vi "BMU诊断标定.vi"(5 "timeout":u32, 6 "Socket":dbl, 7 "通用配置?":bool, 8 "CAN端口":u16(ring), 9 "设备索引号":u16(ring), 10 "CAN卡类型":u32(ring)=21, 11 "从板号":u8=1) -> (3 "成功?":bool)   [LabVIEW 2013] (continued)
                      frame True {
                      }
                    }
                  }
                }
              }
            }
          }
          event "风机继电器": Value Change {
            n2723 = event-data() -> ("NewVal"=w3577:bool)  [unwired: 6 out]
            n2724 = stacked-sequence {
              tunnel: w3577 -> [_ w3590 _]
              frame #0 {
                w3581 = FALSE ("继电器超时处理")
                n2725 = local write "继电器超时处理"(w3581) -> ()
                n2726 = local write "正级继电器 6"(w3581) -> ()
                n2727 = global write "EV05全局变量1.vi" "流控帧"(FALSE ("流控帧")) -> ()
                n2728 = local write "主从选择"(enum32{"主板", "从板"}."主板" ("主从选择")) -> ()
              }
              frame #1 {
                n2729 = case shown="真" w3590 {
                  selector: w3590 -> [w3604 w3624]
                  tunnel: [w3603 w3623] -> w3589
                  tunnel: [w3592 w3612] -> w3584
                  frame True {
                    w3600 = 256.0 ("y")
                    w3592 = u32 1 ("命令序号")
                    w3603 = u8 192 ("命令")
                    n2730 = local read "动作保持时间"() -> (w3601:dbl)
                    n2731 = Quotient & Remainder(x=w3601, y=w3600) -> (x-y*floor(x/y)=w3593:dbl, floor(x/y)=w3597:dbl)
                    n2732 = Quotient & Remainder(x=w3597, y=w3600) -> (x-y*floor(x/y)=w3594:dbl, floor(x/y)=w3598:dbl)
                    n2733 = Quotient & Remainder(x=w3598, y=w3600) -> (x-y*floor(x/y)=w3595:dbl, floor(x/y)=w3599:dbl)
                    n2734 = Boolean To (0,1)(Boolean=w3604) -> (0, 1=w3602:i16)
                    n2735 = local read "设备索引号"() -> (w3609:u16)
                    n2736 = local read "CAN卡类型"() -> (w3610:u32)
                    n2737 = Quotient & Remainder(x=w3599, y=w3600) -> (x-y*floor(x/y)=w3596:dbl)  [unwired: 1 out]
                    n2738 = local read "CAN端口"() -> (w3608:u16)
                    n2739 = Build Array(i16 6 ("元素"), w3602, w3596, w3595, w3594, w3593, 0.0 ("元素")) -> (w3606:dbl[])
                    n2740 = call "多帧发送机制(EV05).vi"("can卡类型"=w3610, "设备索引号"=w3609, "CAN端口"=w3608, "命令"=w3603, "板号"=u8 0, "命令序号"=w3592, "输入数据"=w3606) -> ()  [unwired: 2 in, 11 out]
                  }
                  frame False {
                    w3620 = 256.0 ("y")
                    w3612 = u32 1 ("命令序号")
                    w3623 = u8 192 ("命令")
                    n2741 = local read "动作保持时间"() -> (w3621:dbl)
                    n2742 = Quotient & Remainder(x=w3621, y=w3620) -> (x-y*floor(x/y)=w3613:dbl, floor(x/y)=w3617:dbl)
                    n2743 = Quotient & Remainder(x=w3617, y=w3620) -> (x-y*floor(x/y)=w3614:dbl, floor(x/y)=w3618:dbl)
                    n2744 = Quotient & Remainder(x=w3618, y=w3620) -> (x-y*floor(x/y)=w3615:dbl, floor(x/y)=w3619:dbl)
                    n2745 = Boolean To (0,1)(Boolean=w3624) -> (0, 1=w3622:i16)
                    n2746 = local read "设备索引号"() -> (w3629:u16)
                    n2747 = local read "CAN卡类型"() -> (w3630:u32)
                    n2748 = Quotient & Remainder(x=w3619, y=w3620) -> (x-y*floor(x/y)=w3616:dbl)  [unwired: 1 out]
                    n2749 = local read "CAN端口"() -> (w3628:u16)
                    n2750 = Build Array(i16 6 ("元素"), w3622, w3616, w3615, w3614, w3613, 0.0 ("元素")) -> (w3626:dbl[])
                    n2751 = call "多帧发送机制(EV05).vi"("can卡类型"=w3630, "设备索引号"=w3629, "CAN端口"=w3628, "命令"=w3623, "板号"=u8 0, "命令序号"=w3612, "输入数据"=w3626) -> ()  [unwired: 2 in, 11 out]
                  }
                }
                n2752 = local write "命令序号"(w3584) -> ()
                n2753 = local write "命令"(w3589) -> ()
                n2754 = local write "清BUFF"(FALSE ("清BUFF")) -> ()
                n2755 = local write "控制1"(TRUE ("控制1")) -> ()
                n2756 = global write "EV05全局变量1.vi" "流控帧 2"(TRUE ("流控帧 2")) -> ()
                n2757 = local write "写?"(FALSE ("写?")) -> ()
                n2758 = local write "消除"(TRUE ("消除")) -> ()
              }
              frame #2 {
                n2759 = flat-sequence {
                  tunnel: [w3632] -> w3631
                  tunnel: w3631 -> [w3639]
                  frame #0 {
                    n2760 = while {
                      tunnel: [w3633] -> w3632
                      i -> [w3637]
                      stop <- w3634 stop-if-true
                      n2761 = local read "继电器超时处理"() -> (w3633:bool)
                      n2762 = Greater Or Equal?(x=w3637, y=20) -> (x >= y?=w3635:bool)
                      n2763 = Wait Until Next ms Multiple(millisecond multiple=u32 100 ("毫秒倍数")) -> ()  [unwired: 1 out]
                      n2764 = Or(x=w3633, y=w3635) -> (x .or. y?=w3634:bool)
                    }
                  }
                  frame #1 {
                    n2765 = case shown="假" w3639 {
                      frame False {
                        n2766 = local read "风机继电器"() -> (w3640:bool)
                        n2767 = Not(x=w3640) -> (.not. x?=w3641:bool)
                        n2768 = local write "风机继电器"(w3641) -> ()
                        n2769 = One Button Dialog(message="继电器处理超时" ("消息"), button name ("OK")="是" ("按钮名称（“确定”）")) -> ()  [unwired: 1 out]
                      }
                      frame True {
                      }
                    }
                  }
                }
              }
            }
          }
          event "加热继电器(从)": Value Change {
            n2770 = event-data() -> ("NewVal"=w3644:bool)  [unwired: 6 out]
            n2771 = stacked-sequence {
              tunnel: w3644 -> [_ w3658 _]
              frame #0 {
                w3648 = FALSE ("继电器超时处理")
                n2772 = local write "正级继电器 7"(w3648) -> ()
                n2773 = local write "继电器超时处理"(w3648) -> ()
                n2774 = global write "EV05全局变量1.vi" "流控帧"(FALSE ("流控帧")) -> ()
                n2775 = local write "主从选择"(enum32{"主板", "从板"}."从板" ("主从选择")) -> ()
              }
              frame #1 {
                n2776 = case shown="真" w3658 {
                  selector: w3658 -> [w3673 w3693]
                  tunnel: [w3672 w3692] -> w3657
                  tunnel: [w3671 w3691] -> w3651
                  tunnel: [w3660 w3680] -> w3652
                  frame True {
                    w3668 = 256.0 ("y")
                    w3660 = u32 1 ("命令序号")
                    w3672 = u8 192 ("命令")
                    n2777 = local read "动作保持时间"() -> (w3669:dbl)
                    n2778 = Quotient & Remainder(x=w3669, y=w3668) -> (x-y*floor(x/y)=w3661:dbl, floor(x/y)=w3665:dbl)
                    n2779 = Quotient & Remainder(x=w3665, y=w3668) -> (x-y*floor(x/y)=w3662:dbl, floor(x/y)=w3666:dbl)
                    n2780 = Quotient & Remainder(x=w3666, y=w3668) -> (x-y*floor(x/y)=w3663:dbl, floor(x/y)=w3667:dbl)
                    n2781 = Quotient & Remainder(x=w3667, y=w3668) -> (x-y*floor(x/y)=w3664:dbl)  [unwired: 1 out]
                    n2782 = Boolean To (0,1)(Boolean=w3673) -> (0, 1=w3670:i16)
                    n2783 = local read "设备索引号"() -> (w3677:u16)
                    n2784 = local read "CAN卡类型"() -> (w3678:u32)
                    n2785 = local read "从板板号"() -> (w3671:u8)
                    n2786 = local read "CAN端口"() -> (w3676:u16)
                    n2787 = Build Array(i16 7 ("元素"), w3670, w3664, w3663, w3662, w3661, 0.0 ("元素")) -> (w3675:dbl[])
                    n2788 = call "多帧发送机制(EV05).vi"("can卡类型"=w3678, "设备索引号"=w3677, "CAN端口"=w3676, "命令"=w3672, "板号"=w3671, "命令序号"=w3660, "输入数据"=w3675) -> ()  [unwired: 2 in, 11 out]
                  }
                  frame False {
                    w3688 = 256.0 ("y")
                    w3680 = u32 1 ("命令序号")
                    w3692 = u8 192 ("命令")
                    n2789 = local read "动作保持时间"() -> (w3689:dbl)
                    n2790 = Quotient & Remainder(x=w3689, y=w3688) -> (x-y*floor(x/y)=w3681:dbl, floor(x/y)=w3685:dbl)
                    n2791 = Quotient & Remainder(x=w3685, y=w3688) -> (x-y*floor(x/y)=w3682:dbl, floor(x/y)=w3686:dbl)
                    n2792 = Quotient & Remainder(x=w3686, y=w3688) -> (x-y*floor(x/y)=w3683:dbl, floor(x/y)=w3687:dbl)
                    n2793 = Quotient & Remainder(x=w3687, y=w3688) -> (x-y*floor(x/y)=w3684:dbl)  [unwired: 1 out]
                    n2794 = Boolean To (0,1)(Boolean=w3693) -> (0, 1=w3690:i16)
                    n2795 = local read "设备索引号"() -> (w3697:u16)
                    n2796 = local read "CAN卡类型"() -> (w3698:u32)
                    n2797 = local read "从板板号"() -> (w3691:u8)
                    n2798 = local read "CAN端口"() -> (w3696:u16)
                    n2799 = Build Array(i16 7 ("元素"), w3690, w3684, w3683, w3682, w3681, 0.0 ("元素")) -> (w3695:dbl[])
                    n2800 = call "多帧发送机制(EV05).vi"("can卡类型"=w3698, "设备索引号"=w3697, "CAN端口"=w3696, "命令"=w3692, "板号"=w3691, "命令序号"=w3680, "输入数据"=w3695) -> ()  [unwired: 2 in, 11 out]
                  }
                }
                n2801 = local write "从板板号"(w3651) -> ()
                n2802 = local write "命令序号"(w3652) -> ()
                n2803 = local write "命令"(w3657) -> ()
                n2804 = local write "清BUFF"(FALSE ("清BUFF")) -> ()
                n2805 = local write "写?"(FALSE ("写?")) -> ()
                n2806 = local write "控制1"(TRUE ("控制1")) -> ()
                n2807 = global write "EV05全局变量1.vi" "流控帧 2"(TRUE ("流控帧 2")) -> ()
                n2808 = local write "消除"(TRUE ("消除")) -> ()
              }
              frame #2 {
                n2809 = flat-sequence {
                  tunnel: [w3700] -> w3699
                  tunnel: w3699 -> [w3707]
                  frame #0 {
                    n2810 = while {
                      tunnel: [w3701] -> w3700
                      i -> [w3705]
                      stop <- w3702 stop-if-true
                      n2811 = local read "继电器超时处理"() -> (w3701:bool)
                      n2812 = Greater Or Equal?(x=w3705, y=20) -> (x >= y?=w3703:bool)
                      n2813 = Wait Until Next ms Multiple(millisecond multiple=u32 100 ("毫秒倍数")) -> ()  [unwired: 1 out]
                      n2814 = Or(x=w3701, y=w3703) -> (x .or. y?=w3702:bool)
                    }
                  }
                  frame #1 {
                    n2815 = case shown="假" w3707 {
                      frame False {
                        n2816 = local read "加热继电器(从)"() -> (w3709:bool)
                        n2817 = Not(x=w3709) -> (.not. x?=w3708:bool)
                        n2818 = local write "加热继电器(从)"(w3708) -> ()
                        n2819 = One Button Dialog(message="继电器处理超时" ("消息"), button name ("OK")="是" ("按钮名称（“确定”）")) -> ()  [unwired: 1 out]
                      }
                      frame True {
                      }
                    }
                  }
                }
              }
            }
          }
          event "风机继电器(从)": Value Change {
            n2820 = event-data() -> ("NewVal"=w3712:bool)  [unwired: 6 out]
            n2821 = stacked-sequence {
              tunnel: w3712 -> [_ w3726 _]
              frame #0 {
                w3716 = FALSE ("继电器超时处理")
                n2822 = local write "继电器超时处理"(w3716) -> ()
                n2823 = local write "正级继电器 8"(w3716) -> ()
                n2824 = global write "EV05全局变量1.vi" "流控帧"(FALSE ("流控帧")) -> ()
                n2825 = local write "主从选择"(enum32{"主板", "从板"}."从板" ("主从选择")) -> ()
              }
              frame #1 {
                n2826 = case shown="假" w3726 {
                  selector: w3726 -> [w3741 w3761]
                  tunnel: [w3740 w3760] -> w3725
                  tunnel: [w3739 w3759] -> w3719
                  tunnel: [w3728 w3748] -> w3720
                  frame False {
                    w3736 = 256.0 ("y")
                    w3728 = u32 1 ("命令序号")
                    w3740 = u8 192 ("命令")
                    n2827 = local read "动作保持时间"() -> (w3737:dbl)
                    n2828 = Quotient & Remainder(x=w3737, y=w3736) -> (x-y*floor(x/y)=w3729:dbl, floor(x/y)=w3733:dbl)
                    n2829 = Quotient & Remainder(x=w3733, y=w3736) -> (x-y*floor(x/y)=w3730:dbl, floor(x/y)=w3734:dbl)
                    n2830 = Quotient & Remainder(x=w3734, y=w3736) -> (x-y*floor(x/y)=w3731:dbl, floor(x/y)=w3735:dbl)
                    n2831 = Quotient & Remainder(x=w3735, y=w3736) -> (x-y*floor(x/y)=w3732:dbl)  [unwired: 1 out]
                    n2832 = local read "设备索引号"() -> (w3745:u16)
                    n2833 = local read "CAN卡类型"() -> (w3746:u32)
                    n2834 = local read "从板板号"() -> (w3739:u8)
                    n2835 = Boolean To (0,1)(Boolean=w3741) -> (0, 1=w3738:i16)
                    n2836 = local read "CAN端口"() -> (w3744:u16)
                    n2837 = Build Array(i16 8 ("元素"), w3738, w3732, w3731, w3730, w3729, 0.0 ("元素")) -> (w3743:dbl[])
                    n2838 = call "多帧发送机制(EV05).vi"("can卡类型"=w3746, "设备索引号"=w3745, "CAN端口"=w3744, "命令"=w3740, "板号"=w3739, "命令序号"=w3728, "输入数据"=w3743) -> ()  [unwired: 2 in, 11 out]
                  }
                  frame True {
                    w3756 = 256.0 ("y")
                    w3748 = u32 1 ("命令序号")
                    w3760 = u8 192 ("命令")
                    n2839 = local read "动作保持时间"() -> (w3757:dbl)
                    n2840 = Quotient & Remainder(x=w3757, y=w3756) -> (x-y*floor(x/y)=w3749:dbl, floor(x/y)=w3753:dbl)
                    n2841 = Quotient & Remainder(x=w3753, y=w3756) -> (x-y*floor(x/y)=w3750:dbl, floor(x/y)=w3754:dbl)
                    n2842 = Quotient & Remainder(x=w3754, y=w3756) -> (x-y*floor(x/y)=w3751:dbl, floor(x/y)=w3755:dbl)
                    n2843 = Quotient & Remainder(x=w3755, y=w3756) -> (x-y*floor(x/y)=w3752:dbl)  [unwired: 1 out]
                    n2844 = local read "设备索引号"() -> (w3765:u16)
                    n2845 = local read "CAN卡类型"() -> (w3766:u32)
                    n2846 = local read "从板板号"() -> (w3759:u8)
                    n2847 = Boolean To (0,1)(Boolean=w3761) -> (0, 1=w3758:i16)
                    n2848 = local read "CAN端口"() -> (w3764:u16)
                    n2849 = Build Array(i16 8 ("元素"), w3758, w3752, w3751, w3750, w3749, 0.0 ("元素")) -> (w3763:dbl[])
                    n2850 = call "多帧发送机制(EV05).vi"("can卡类型"=w3766, "设备索引号"=w3765, "CAN端口"=w3764, "命令"=w3760, "板号"=w3759, "命令序号"=w3748, "输入数据"=w3763) -> ()  [unwired: 2 in, 11 out]
                  }
                }
                n2851 = local write "从板板号"(w3719) -> ()
                n2852 = local write "清BUFF"(FALSE ("清BUFF")) -> ()
                n2853 = local write "命令序号"(w3720) -> ()
                n2854 = local write "命令"(w3725) -> ()
                n2855 = local write "控制1"(TRUE ("控制1")) -> ()
                n2856 = local write "写?"(FALSE ("写?")) -> ()
                n2857 = local write "消除"(TRUE ("消除")) -> ()
                n2858 = global write "EV05全局变量1.vi" "流控帧 2"(TRUE ("流控帧 2")) -> ()
              }
              frame #2 {
                n2859 = flat-sequence {
                  tunnel: [w3768] -> w3767
                  tunnel: w3767 -> [w3775]
                  frame #0 {
                    n2860 = while {
                      tunnel: [w3769] -> w3768
                      i -> [w3773]
                      stop <- w3770 stop-if-true
                      n2861 = local read "继电器超时处理"() -> (w3769:bool)
                      n2862 = Greater Or Equal?(x=w3773, y=20) -> (x >= y?=w3771:bool)
                      n2863 = Wait Until Next ms Multiple(millisecond multiple=u32 100 ("毫秒倍数")) -> ()  [unwired: 1 out]
                      n2864 = Or(x=w3769, y=w3771) -> (x .or. y?=w3770:bool)
                    }
                  }
                  frame #1 {
                    n2865 = case shown="假" w3775 {
                      frame False {
                        n2866 = local read "风机继电器(从)"() -> (w3777:bool)
                        n2867 = Not(x=w3777) -> (.not. x?=w3776:bool)
                        n2868 = local write "风机继电器(从)"(w3776) -> ()
                        n2869 = One Button Dialog(message="继电器处理超时" ("消息"), button name ("OK")="是" ("按钮名称（“确定”）")) -> ()  [unwired: 1 out]
                      }
                      frame True {
                      }
                    }
                  }
                }
              }
            }
          }
          event "DO1": Value Change {
            n2870 = event-data() -> ("NewVal"=w3780:bool)  [unwired: 6 out]
            n2871 = stacked-sequence {
              tunnel: w3780 -> [_ w3793 _]
              frame #0 {
                w3783 = FALSE ("清BUFF")
                n2872 = local write "继电器超时处理"(FALSE ("继电器超时处理")) -> ()
                n2873 = local write "清BUFF"(w3783) -> ()
                n2874 = local write "正级继电器 9"(w3783) -> ()
                n2875 = local write "主从选择"(enum32{"主板", "从板"}."主板" ("主从选择")) -> ()
              }
              frame #1 {
                n2876 = case shown="真" w3793 {
                  selector: w3793 -> [w3808 w3828]
                  tunnel: [w3807 w3827] -> w3792
                  tunnel: [w3795 w3815] -> w3787
                  frame False {
                    w3803 = 256.0 ("y")
                    w3795 = u32 2 ("命令序号")
                    w3807 = u8 192 ("命令")
                    n2877 = local read "动作保持时间"() -> (w3804:dbl)
                    n2878 = Quotient & Remainder(x=w3804, y=w3803) -> (x-y*floor(x/y)=w3796:dbl, floor(x/y)=w3800:dbl)
                    n2879 = Quotient & Remainder(x=w3800, y=w3803) -> (x-y*floor(x/y)=w3797:dbl, floor(x/y)=w3801:dbl)
                    n2880 = Quotient & Remainder(x=w3801, y=w3803) -> (x-y*floor(x/y)=w3798:dbl, floor(x/y)=w3802:dbl)
                    n2881 = local read "设备索引号"() -> (w3812:u16)
                    n2882 = local read "CAN卡类型"() -> (w3813:u32)
                    n2883 = local read "CAN端口"() -> (w3811:u16)
                    n2884 = Boolean To (0,1)(Boolean=w3808) -> (0, 1=w3805:i16)
                    n2885 = Quotient & Remainder(x=w3802, y=w3803) -> (x-y*floor(x/y)=w3799:dbl)  [unwired: 1 out]
                    n2886 = Build Array(i16 1 ("元素"), w3805, w3799, w3798, w3797, w3796, 0.0 ("元素")) -> (w3809:dbl[])
                    n2887 = call "多帧发送机制(EV05).vi"("can卡类型"=w3813, "设备索引号"=w3812, "CAN端口"=w3811, "命令"=w3807, "板号"=u8 0, "命令序号"=w3795, "输入数据"=w3809) -> ()  [unwired: 2 in, 11 out]
                  }
                  frame True {
                    w3823 = 256.0 ("y")
                    w3815 = u32 2 ("命令序号")
                    w3827 = u8 192 ("命令")
                    n2888 = local read "动作保持时间"() -> (w3824:dbl)
                    n2889 = Quotient & Remainder(x=w3824, y=w3823) -> (x-y*floor(x/y)=w3816:dbl, floor(x/y)=w3820:dbl)
                    n2890 = Quotient & Remainder(x=w3820, y=w3823) -> (x-y*floor(x/y)=w3817:dbl, floor(x/y)=w3821:dbl)
                    n2891 = Quotient & Remainder(x=w3821, y=w3823) -> (x-y*floor(x/y)=w3818:dbl, floor(x/y)=w3822:dbl)
                    n2892 = local read "设备索引号"() -> (w3832:u16)
                    n2893 = local read "CAN卡类型"() -> (w3833:u32)
                    n2894 = local read "CAN端口"() -> (w3831:u16)
                    n2895 = Boolean To (0,1)(Boolean=w3828) -> (0, 1=w3825:i16)
                    n2896 = Quotient & Remainder(x=w3822, y=w3823) -> (x-y*floor(x/y)=w3819:dbl)  [unwired: 1 out]
                    n2897 = Build Array(i16 1 ("元素"), w3825, w3819, w3818, w3817, w3816, 0.0 ("元素")) -> (w3829:dbl[])
                    n2898 = call "多帧发送机制(EV05).vi"("can卡类型"=w3833, "设备索引号"=w3832, "CAN端口"=w3831, "命令"=w3827, "板号"=u8 0, "命令序号"=w3815, "输入数据"=w3829) -> ()  [unwired: 2 in, 11 out]
                  }
                }
                n2899 = local write "命令序号"(w3787) -> ()
                n2900 = local write "命令"(w3792) -> ()
                n2901 = local write "控制1"(TRUE ("控制1")) -> ()
                n2902 = local write "写?"(FALSE ("写?")) -> ()
                n2903 = local write "消除"(TRUE ("消除")) -> ()
                n2904 = global write "EV05全局变量1.vi" "流控帧 2"(TRUE ("流控帧 2")) -> ()
                n2905 = global write "EV05全局变量1.vi" "流控帧"(FALSE ("流控帧")) -> ()
              }
              frame #2 {
                n2906 = flat-sequence {
                  tunnel: [w3835] -> w3834
                  tunnel: w3834 -> [w3842]
                  frame #0 {
                    n2907 = while {
                      tunnel: [w3836] -> w3835
                      i -> [w3840]
                      stop <- w3837 stop-if-true
                      n2908 = local read "继电器超时处理"() -> (w3836:bool)
                      n2909 = Greater Or Equal?(x=w3840, y=20) -> (x >= y?=w3838:bool)
                      n2910 = Wait Until Next ms Multiple(millisecond multiple=u32 100 ("毫秒倍数")) -> ()  [unwired: 1 out]
                      n2911 = Or(x=w3836, y=w3838) -> (x .or. y?=w3837:bool)
                    }
                  }
                  frame #1 {
                    n2912 = case shown="假" w3842 {
                      frame False {
                        n2913 = local read "DO1"() -> (w3844:bool)
                        n2914 = Not(x=w3844) -> (.not. x?=w3843:bool)
                        n2915 = local write "DO1"(w3843) -> ()
                        n2916 = One Button Dialog(message="DO控制处理超时" ("消息"), button name ("OK")="是" ("按钮名称（“确定”）")) -> ()  [unwired: 1 out]
                      }
                      frame True {
                      }
                    }
                  }
                }
              }
            }
          }
          event "DO2": Value Change {
            n2917 = event-data() -> ("NewVal"=w3847:bool)  [unwired: 6 out]
            n2918 = stacked-sequence {
              tunnel: w3847 -> [_ w3860 _]
              frame #0 {
                w3850 = FALSE ("清BUFF")
                n2919 = local write "继电器超时处理"(FALSE ("继电器超时处理")) -> ()
                n2920 = local write "主从选择"(enum32{"主板", "从板"}."主板" ("主从选择")) -> ()
                n2921 = local write "清BUFF"(w3850) -> ()
                n2922 = local write "正级继电器 10"(w3850) -> ()
              }
              frame #1 {
                n2923 = case shown="真" w3860 {
                  selector: w3860 -> [w3875 w3895]
                  tunnel: [w3874 w3894] -> w3859
                  tunnel: [w3862 w3882] -> w3854
                  frame False {
                    w3870 = 256.0 ("y")
                    w3862 = u32 2 ("命令序号")
                    w3874 = u8 192 ("命令")
                    n2924 = local read "动作保持时间"() -> (w3871:dbl)
                    n2925 = Quotient & Remainder(x=w3871, y=w3870) -> (x-y*floor(x/y)=w3863:dbl, floor(x/y)=w3867:dbl)
                    n2926 = Quotient & Remainder(x=w3867, y=w3870) -> (x-y*floor(x/y)=w3864:dbl, floor(x/y)=w3868:dbl)
                    n2927 = Quotient & Remainder(x=w3868, y=w3870) -> (x-y*floor(x/y)=w3865:dbl, floor(x/y)=w3869:dbl)
                    n2928 = local read "设备索引号"() -> (w3879:u16)
                    n2929 = local read "CAN卡类型"() -> (w3880:u32)
                    n2930 = local read "CAN端口"() -> (w3878:u16)
                    n2931 = Boolean To (0,1)(Boolean=w3875) -> (0, 1=w3872:i16)
                    n2932 = Quotient & Remainder(x=w3869, y=w3870) -> (x-y*floor(x/y)=w3866:dbl)  [unwired: 1 out]
                    n2933 = Build Array(i16 2 ("元素"), w3872, w3866, w3865, w3864, w3863, 0.0 ("元素")) -> (w3876:dbl[])
                    n2934 = call "多帧发送机制(EV05).vi"("can卡类型"=w3880, "设备索引号"=w3879, "CAN端口"=w3878, "命令"=w3874, "板号"=u8 0, "命令序号"=w3862, "输入数据"=w3876) -> ()  [unwired: 2 in, 11 out]
                  }
                  frame True {
                    w3890 = 256.0 ("y")
                    w3882 = u32 2 ("命令序号")
                    w3894 = u8 192 ("命令")
                    n2935 = local read "动作保持时间"() -> (w3891:dbl)
                    n2936 = Quotient & Remainder(x=w3891, y=w3890) -> (x-y*floor(x/y)=w3883:dbl, floor(x/y)=w3887:dbl)
                    n2937 = Quotient & Remainder(x=w3887, y=w3890) -> (x-y*floor(x/y)=w3884:dbl, floor(x/y)=w3888:dbl)
                    n2938 = Quotient & Remainder(x=w3888, y=w3890) -> (x-y*floor(x/y)=w3885:dbl, floor(x/y)=w3889:dbl)
                    n2939 = local read "设备索引号"() -> (w3899:u16)
                    n2940 = local read "CAN卡类型"() -> (w3900:u32)
                    n2941 = local read "CAN端口"() -> (w3898:u16)
                    n2942 = Boolean To (0,1)(Boolean=w3895) -> (0, 1=w3892:i16)
                    n2943 = Quotient & Remainder(x=w3889, y=w3890) -> (x-y*floor(x/y)=w3886:dbl)  [unwired: 1 out]
                    n2944 = Build Array(i16 2 ("元素"), w3892, w3886, w3885, w3884, w3883, 0.0 ("元素")) -> (w3896:dbl[])
                    n2945 = call "多帧发送机制(EV05).vi"("can卡类型"=w3900, "设备索引号"=w3899, "CAN端口"=w3898, "命令"=w3894, "板号"=u8 0, "命令序号"=w3882, "输入数据"=w3896) -> ()  [unwired: 2 in, 11 out]
                  }
                }
                n2946 = local write "命令序号"(w3854) -> ()
                n2947 = local write "命令"(w3859) -> ()
                n2948 = local write "控制1"(TRUE ("控制1")) -> ()
                n2949 = local write "写?"(FALSE ("写?")) -> ()
                n2950 = local write "消除"(TRUE ("消除")) -> ()
                n2951 = global write "EV05全局变量1.vi" "流控帧 2"(TRUE ("流控帧 2")) -> ()
                n2952 = global write "EV05全局变量1.vi" "流控帧"(FALSE ("流控帧")) -> ()
              }
              frame #2 {
                n2953 = flat-sequence {
                  tunnel: [w3902] -> w3901
                  tunnel: w3901 -> [w3909]
                  frame #0 {
                    n2954 = while {
                      tunnel: [w3903] -> w3902
                      i -> [w3907]
                      stop <- w3904 stop-if-true
                      n2955 = local read "继电器超时处理"() -> (w3903:bool)
                      n2956 = Greater Or Equal?(x=w3907, y=20) -> (x >= y?=w3905:bool)
                      n2957 = Wait Until Next ms Multiple(millisecond multiple=u32 100 ("毫秒倍数")) -> ()  [unwired: 1 out]
                      n2958 = Or(x=w3903, y=w3905) -> (x .or. y?=w3904:bool)
                    }
                  }
                  frame #1 {
                    n2959 = case shown="假" w3909 {
                      frame False {
                        n2960 = local read "DO2"() -> (w3911:bool)
                        n2961 = Not(x=w3911) -> (.not. x?=w3910:bool)
                        n2962 = local write "DO2"(w3910) -> ()
                        n2963 = One Button Dialog(message="DO控制处理超时" ("消息"), button name ("OK")="是" ("按钮名称（“确定”）")) -> ()  [unwired: 1 out]
                      }
                      frame True {
                      }
                    }
                  }
                }
              }
            }
          }
          event "DO1 2": Value Change {
            n2964 = event-data() -> ("NewVal"=w3914:bool)  [unwired: 6 out]
            n2965 = stacked-sequence {
              tunnel: w3914 -> [_ w3928 _]
              frame #0 {
                w3917 = FALSE ("继电器超时处理")
                n2966 = local write "继电器超时处理"(w3917) -> ()
                n2967 = local write "正级继电器 11"(w3917) -> ()
                n2968 = local write "主从选择"(enum32{"主板", "从板"}."从板" ("主从选择")) -> ()
              }
              frame #1 {
                n2969 = case shown="假" w3928 {
                  selector: w3928 -> [w3943 w3963]
                  tunnel: [w3942 w3962] -> w3927
                  tunnel: [w3941 w3961] -> w3921
                  tunnel: [w3930 w3950] -> w3922
                  frame True {
                    w3938 = 256.0 ("y")
                    w3930 = u32 2 ("命令序号")
                    w3942 = u8 192 ("命令")
                    n2970 = local read "动作保持时间"() -> (w3939:dbl)
                    n2971 = Quotient & Remainder(x=w3939, y=w3938) -> (x-y*floor(x/y)=w3931:dbl, floor(x/y)=w3935:dbl)
                    n2972 = Quotient & Remainder(x=w3935, y=w3938) -> (x-y*floor(x/y)=w3932:dbl, floor(x/y)=w3936:dbl)
                    n2973 = Quotient & Remainder(x=w3936, y=w3938) -> (x-y*floor(x/y)=w3933:dbl, floor(x/y)=w3937:dbl)
                    n2974 = Quotient & Remainder(x=w3937, y=w3938) -> (x-y*floor(x/y)=w3934:dbl)  [unwired: 1 out]
                    n2975 = Boolean To (0,1)(Boolean=w3943) -> (0, 1=w3940:i16)
                    n2976 = local read "设备索引号"() -> (w3947:u16)
                    n2977 = local read "CAN卡类型"() -> (w3948:u32)
                    n2978 = local read "从板板号"() -> (w3941:u8)
                    n2979 = local read "CAN端口"() -> (w3946:u16)
                    n2980 = Build Array(i16 3 ("元素"), w3940, w3934, w3933, w3932, w3931, 0.0 ("元素")) -> (w3945:dbl[])
                    n2981 = call "多帧发送机制(EV05).vi"("can卡类型"=w3948, "设备索引号"=w3947, "CAN端口"=w3946, "命令"=w3942, "板号"=w3941, "命令序号"=w3930, "输入数据"=w3945) -> ()  [unwired: 2 in, 11 out]
                  }
                  frame False {
                    w3958 = 256.0 ("y")
                    w3950 = u32 2 ("命令序号")
                    w3962 = u8 192 ("命令")
                    n2982 = local read "动作保持时间"() -> (w3959:dbl)
                    n2983 = Quotient & Remainder(x=w3959, y=w3958) -> (x-y*floor(x/y)=w3951:dbl, floor(x/y)=w3955:dbl)
                    n2984 = Quotient & Remainder(x=w3955, y=w3958) -> (x-y*floor(x/y)=w3952:dbl, floor(x/y)=w3956:dbl)
                    n2985 = Quotient & Remainder(x=w3956, y=w3958) -> (x-y*floor(x/y)=w3953:dbl, floor(x/y)=w3957:dbl)
                    n2986 = Quotient & Remainder(x=w3957, y=w3958) -> (x-y*floor(x/y)=w3954:dbl)  [unwired: 1 out]
                    n2987 = Boolean To (0,1)(Boolean=w3963) -> (0, 1=w3960:i16)
                    n2988 = local read "设备索引号"() -> (w3967:u16)
                    n2989 = local read "CAN卡类型"() -> (w3968:u32)
                    n2990 = local read "从板板号"() -> (w3961:u8)
                    n2991 = local read "CAN端口"() -> (w3966:u16)
                    n2992 = Build Array(i16 1 ("元素"), w3960, w3954, w3953, w3952, w3951, 0.0 ("元素")) -> (w3965:dbl[])
                    n2993 = call "多帧发送机制(EV05).vi"("can卡类型"=w3968, "设备索引号"=w3967, "CAN端口"=w3966, "命令"=w3962, "板号"=w3961, "命令序号"=w3950, "输入数据"=w3965) -> ()  [unwired: 2 in, 11 out]
                  }
                }
                n2994 = local write "从板板号"(w3921) -> ()
                n2995 = local write "命令序号"(w3922) -> ()
                n2996 = local write "命令"(w3927) -> ()
                n2997 = local write "清BUFF"(FALSE ("清BUFF")) -> ()
                n2998 = local write "写?"(FALSE ("写?")) -> ()
                n2999 = local write "控制1"(TRUE ("控制1")) -> ()
                n3000 = global write "EV05全局变量1.vi" "流控帧"(FALSE ("流控帧")) -> ()
                n3001 = global write "EV05全局变量1.vi" "流控帧 2"(TRUE ("流控帧 2")) -> ()
                n3002 = local write "消除"(TRUE ("消除")) -> ()
              }
              frame #2 {
                n3003 = flat-sequence {
                  tunnel: [w3970] -> w3969
                  tunnel: w3969 -> [w3977]
                  frame #0 {
                    n3004 = while {
                      tunnel: [w3971] -> w3970
                      i -> [w3975]
                      stop <- w3972 stop-if-true
                      n3005 = local read "继电器超时处理"() -> (w3971:bool)
                      n3006 = Greater Or Equal?(x=w3975, y=20) -> (x >= y?=w3973:bool)
                      n3007 = Wait Until Next ms Multiple(millisecond multiple=u32 100 ("毫秒倍数")) -> ()  [unwired: 1 out]
                      n3008 = Or(x=w3971, y=w3973) -> (x .or. y?=w3972:bool)
                    }
                  }
                  frame #1 {
                    n3009 = case shown="假" w3977 {
                      frame False {
                        n3010 = local read "DO1 2"() -> (w3979:bool)
                        n3011 = Not(x=w3979) -> (.not. x?=w3978:bool)
                        n3012 = local write "DO1 2"(w3978) -> ()
                        n3013 = One Button Dialog(message="DO控制处理超时" ("消息"), button name ("OK")="是" ("按钮名称（“确定”）")) -> ()  [unwired: 1 out]
                      }
                      frame True {
                      }
                    }
                  }
                }
              }
            }
          }
          event "读取转换为写入": Value Change {
            n3014 = event-data() -> ("NewVal"=w3982:bool)  [unwired: 6 out]
            n3015 = case shown="真" w3982 {
              tunnel: w3986 -> [w3988 w3993]
              tunnel: [w3988 w3992] -> w3985
              tunnel: w3984 -> [w3987 w3991]
              tunnel: [w3987 w3990] -> w3983
              frame False {
              }
              frame True {
                n3016 = Enqueue Element(queue=w3993, element="读取转换为写入", error in (no error)=w3991) -> (queue out=w3992:refnum<queue>, error out=w3990:errorcluster)  [unwired: 2 out]
              }
            }
          }
          event "读取故障详细状态": Value Change {
            n3017 = event-data() -> ("NewVal"=w3998:bool)  [unwired: 5 out]
            n3018 = case shown="真" w3998 {
              tunnel: w3997 -> [w4000 w4013]
              tunnel: w3996 -> [w3999 w4012]
              tunnel: [w4000 w4011] -> w3995
              tunnel: [w3999 w4010] -> w3994
              frame False {
              }
              frame True {
                n3019 = disable-structure shown="启用" {
                  disable-tunnel: [w4022 TRUE ("发送成功")] -> w4009
                  frame Disabled {
                    n3020 = local read "主从选择"() -> (w4014:enum32{"主板", "从板"})
                    n3021 = case shown="\"主板\", 默认" w4014 {
                      tunnel: [0.0 ("FUNC") w4024] -> w4019
                      frame "主板", Default {
                      }
                      frame "从板" {
                        n3022 = local read "从板号"() -> (w4024:u8)
                      }
                    }
                    n3023 = local read "设备索引号"() -> (w4016:u16)
                    n3024 = local read "CAN卡类型"() -> (w4017:u32)
                    n3025 = local read "CAN端口"() -> (w4015:u16)
                    n3026 = call "标定授权发送.vi"("CAN卡类型"=w4017, "解锁类型"=enum16{"读取", "写", "下载"}."写", "设备索引号"=w4016, "CAN端口"=w4015, "是否连接"=TRUE, "板选择"=0, "FUNC"=w4019) -> ("发送成功"=w4022:bool)  [unwired: 8 out]
                  }
                  frame Enabled {
                  }
                }
                n3027 = case shown="真" w4009 {
                  tunnel: w4013 -> [w4027 w4032]
                  tunnel: w4012 -> [w4026 w4031]
                  tunnel: [w4027 w4029] -> w4011
                  tunnel: [w4026 w4028] -> w4010
                  frame False {
                  }
                  frame True {
                    n3028 = Enqueue Element(queue=w4032, element="读取故障状态" ("元素"), error in (no error)=w4031) -> (queue out=w4029:refnum<queue>, error out=w4028:errorcluster)  [unwired: 2 out]
                  }
                }
                n3029 = local write "电池故障"(string[][] []) -> ()
                n3030 = global write "EV05全局变量1.vi" "流控帧 2"(TRUE ("流控帧")) -> ()
                n3031 = local write "写?"(FALSE ("写?")) -> ()
                n3032 = local write "控制1"(TRUE ("控制1")) -> ()
                n3033 = local write "消除"(TRUE ("消除")) -> ()
                n3034 = local write "清BUFF"(FALSE ("清BUFF")) -> ()
                n3035 = global write "EV05全局变量1.vi" "流控帧"(FALSE ("流控帧")) -> ()
                n3036 = call <vilib>:"Set Busy.vi"("disable click? (T)"=FALSE) -> ()  [unwired: 3 in, 8 out]
              }
            }
          }
          event "项目软本读取": Value Change {
            n3037 = event-data() -> ("NewVal"=w4037:bool)  [unwired: 5 out]
            n3038 = case shown="真" w4037 {
              tunnel: w4036 -> [w4039 w4046]
              tunnel: w4035 -> [w4038 w4045]
              tunnel: [w4039 w4044] -> w4034
              tunnel: [w4038 w4043] -> w4033
              frame False {
              }
              frame True {
                n3039 = global read "EV05全局变量1.vi" "授权功能"() -> (w4041:bool)
                n3040 = case shown="假" w4041 {
                  tunnel: [TRUE ("发送成功") w4065] -> w4042
                  frame False {
                  }
                  frame True {
                    n3041 = local read "设备索引号"() -> (w4060:u16)
                    n3042 = local read "CAN卡类型"() -> (w4061:u32)
                    n3043 = local read "CAN端口"() -> (w4059:u16)
                    n3044 = call "标定授权发送.vi"("CAN卡类型"=w4061, "解锁类型"=enum16{"读取", "写", "下载"}."读取", "设备索引号"=w4060, "CAN端口"=w4059, "是否连接"=TRUE, "板选择"=0, "FUNC"=u32 0) -> ("发送成功"=w4065:bool)  [unwired: 8 out]
                  }
                }
                n3045 = stacked-sequence {
                  tunnel: [w4049] -> w4040
                  frame #0 {
                    w4049 = FALSE ("disable click? (T)")
                    w4052 = FALSE ("写?")
                    n3046 = local write "写?"(w4052) -> ()
                    n3047 = global write "EV05全局变量1.vi" "写入超时"(w4052) -> ()
                    n3048 = local write "项目软件版本号"(" " ("项目软件版本号")) -> ()
                    n3049 = global write "EV05全局变量1.vi" "流控帧"(FALSE ("流控帧")) -> ()
                    n3050 = local write "主从选择"(enum32{"主板", "从板"}."主板" ("主从选择")) -> ()
                    n3051 = call <vilib>:"Set Busy.vi"("disable click? (T)"=w4049) -> ()  [unwired: 3 in, 8 out]
                    n3052 = local write "清BUFF"(FALSE ("清BUFF")) -> ()
                    n3053 = property on="保存版本信息" class="Bool (严格)"("Visible"=TRUE ("可见")) -> ()  [unwired: 2 in, 2 out]
                    n3054 = global write "EV05全局变量1.vi" "流控帧 2"(TRUE ("流控帧 2")) -> ()
                    n3055 = local write "控制1"(TRUE ("控制1")) -> ()
                    n3056 = local write "消除"(TRUE ("消除")) -> ()
                  }
                }
                n3057 = case shown="真" w4042 {
                  tunnel: w4046 -> [w4067 w4072]
                  tunnel: w4045 -> [w4066 w4071]
                  tunnel: [w4067 w4069] -> w4044
                  tunnel: [w4066 w4068] -> w4043
                  tunnel: w4040 -> [_ _]
                  frame False {
                  }
                  frame True {
                    n3058 = Enqueue Element(queue=w4072, element="项目软件版本读取" ("元素"), error in (no error)=w4071) -> (queue out=w4069:refnum<queue>, error out=w4068:errorcluster)  [unwired: 2 out]
                  }
                }
              }
            }
          }
          event "读硬件版本号": Value Change {
            n3059 = event-data() -> ("NewVal"=w4077:bool)  [unwired: 5 out]
            n3060 = case shown="真" w4077 {
              tunnel: w4076 -> [w4079 w4086]
              tunnel: w4075 -> [w4078 w4085]
              tunnel: [w4079 w4084] -> w4074
              tunnel: [w4078 w4083] -> w4073
              frame False {
              }
              frame True {
                n3061 = global read "EV05全局变量1.vi" "授权功能"() -> (w4081:bool)
                n3062 = case shown="假" w4081 {
                  tunnel: [TRUE ("发送成功") w4105] -> w4082
                  frame False {
                  }
                  frame True {
                    n3063 = local read "设备索引号"() -> (w4100:u16)
                    n3064 = local read "CAN卡类型"() -> (w4101:u32)
                    n3065 = local read "CAN端口"() -> (w4099:u16)
                    n3066 = call "标定授权发送.vi"("CAN卡类型"=w4101, "解锁类型"=enum16{"读取", "写", "下载"}."读取", "设备索引号"=w4100, "CAN端口"=w4099, "是否连接"=TRUE, "板选择"=0, "FUNC"=u32 0) -> ("发送成功"=w4105:bool)  [unwired: 8 out]
                  }
                }
                n3067 = stacked-sequence {
                  tunnel: [w4089] -> w4080
                  frame #0 {
                    w4089 = TRUE ("控制1")
                    w4093 = FALSE ("写?")
                    n3068 = local write "写?"(w4093) -> ()
                    n3069 = global write "EV05全局变量1.vi" "写入超时"(w4093) -> ()
                    n3070 = call <vilib>:"Set Busy.vi"("disable click? (T)"=FALSE) -> ()  [unwired: 3 in, 8 out]
                    n3071 = local write "硬件版本号"("" ("硬件版本号")) -> ()
                    n3072 = property on="保存版本信息" class="Bool (严格)"("Visible"=TRUE ("可见")) -> ()  [unwired: 2 in, 2 out]
                    n3073 = local write "主从选择"(enum32{"主板", "从板"}."主板" ("主从选择")) -> ()
                    n3074 = local write "控制1"(w4089) -> ()
                    n3075 = local write "清BUFF"(FALSE ("清BUFF")) -> ()
                    n3076 = global write "EV05全局变量1.vi" "流控帧 2"(TRUE ("流控帧 2")) -> ()
                    n3077 = local write "消除"(TRUE ("消除")) -> ()
                    n3078 = global write "EV05全局变量1.vi" "流控帧"(FALSE ("流控帧")) -> ()
                  }
                }
                n3079 = case shown="真" w4082 {
                  tunnel: w4086 -> [w4107 w4112]
                  tunnel: w4085 -> [w4106 w4111]
                  tunnel: [w4107 w4109] -> w4084
                  tunnel: [w4106 w4108] -> w4083
                  tunnel: w4080 -> [_ _]
                  frame False {
                  }
                  frame True {
                    n3080 = Enqueue Element(queue=w4112, element="硬件版本读取" ("元素"), error in (no error)=w4111) -> (queue out=w4109:refnum<queue>, error out=w4108:errorcluster)  [unwired: 2 out]
                  }
                }
              }
            }
          }
          event "平台软件版本读取": Value Change {
            n3081 = event-data() -> ("NewVal"=w4117:bool)  [unwired: 5 out]
            n3082 = case shown="真" w4117 {
              tunnel: w4116 -> [w4119 w4126]
              tunnel: w4115 -> [w4118 w4125]
              tunnel: [w4119 w4124] -> w4114
              tunnel: [w4118 w4123] -> w4113
              frame False {
              }
              frame True {
                n3083 = global read "EV05全局变量1.vi" "授权功能"() -> (w4121:bool)
                n3084 = case shown="假" w4121 {
                  tunnel: [TRUE ("发送成功") w4145] -> w4122
                  frame False {
                  }
                  frame True {
                    n3085 = local read "设备索引号"() -> (w4140:u16)
                    n3086 = local read "CAN卡类型"() -> (w4141:u32)
                    n3087 = local read "CAN端口"() -> (w4139:u16)
                    n3088 = call "标定授权发送.vi"("CAN卡类型"=w4141, "解锁类型"=enum16{"读取", "写", "下载"}."读取", "设备索引号"=w4140, "CAN端口"=w4139, "是否连接"=TRUE, "板选择"=0, "FUNC"=u32 0) -> ("发送成功"=w4145:bool)  [unwired: 8 out]
                  }
                }
                n3089 = stacked-sequence {
                  tunnel: [w4129] -> w4120
                  frame #0 {
                    w4129 = TRUE ("控制1")
                    w4133 = FALSE ("写?")
                    n3090 = call <vilib>:"Set Busy.vi"("disable click? (T)"=FALSE) -> ()  [unwired: 3 in, 8 out]
                    n3091 = local write "写?"(w4133) -> ()
                    n3092 = global write "EV05全局变量1.vi" "写入超时"(w4133) -> ()
                    n3093 = local write "平台软件版本号"(" " ("平台软件版本号")) -> ()
                    n3094 = local write "控制1"(w4129) -> ()
                    n3095 = local write "消除"(TRUE ("消除")) -> ()
                    n3096 = property on="保存版本信息" class="Bool (严格)"("Visible"=TRUE ("可见")) -> ()  [unwired: 2 in, 2 out]
                    n3097 = global write "EV05全局变量1.vi" "流控帧 2"(TRUE ("流控帧 2")) -> ()
                    n3098 = local write "主从选择"(enum32{"主板", "从板"}."主板" ("主从选择")) -> ()
                    n3099 = local write "清BUFF"(FALSE ("清BUFF")) -> ()
                    n3100 = global write "EV05全局变量1.vi" "流控帧"(FALSE ("流控帧")) -> ()
                  }
                }
                n3101 = case shown="真" w4122 {
                  tunnel: w4126 -> [w4147 w4152]
                  tunnel: w4125 -> [w4146 w4151]
                  tunnel: [w4147 w4149] -> w4124
                  tunnel: [w4146 w4148] -> w4123
                  tunnel: w4120 -> [_ _]
                  frame False {
                  }
                  frame True {
                    n3102 = Enqueue Element(queue=w4152, element="平台软件版本读取" ("元素"), error in (no error)=w4151) -> (queue out=w4149:refnum<queue>, error out=w4148:errorcluster)  [unwired: 2 out]
                  }
                }
              }
            }
          }
          event "模块版本读取": Value Change {
            n3103 = event-data() -> ("NewVal"=w4157:bool)  [unwired: 5 out]
            n3104 = case shown="真" w4157 {
              tunnel: w4156 -> [w4159 w4166]
              tunnel: w4155 -> [w4158 w4165]
              tunnel: [w4159 w4164] -> w4154
              tunnel: [w4158 w4163] -> w4153
              frame False {
              }
              frame True {
                n3105 = global read "EV05全局变量1.vi" "授权功能"() -> (w4161:bool)
                n3106 = case shown="假" w4161 {
                  tunnel: [TRUE ("发送成功") w4184] -> w4162
                  frame False {
                  }
                  frame True {
                    n3107 = local read "设备索引号"() -> (w4179:u16)
                    n3108 = local read "CAN卡类型"() -> (w4180:u32)
                    n3109 = local read "CAN端口"() -> (w4178:u16)
                    n3110 = call "标定授权发送.vi"("CAN卡类型"=w4180, "解锁类型"=enum16{"读取", "写", "下载"}."读取", "设备索引号"=w4179, "CAN端口"=w4178, "是否连接"=TRUE, "板选择"=0, "FUNC"=u32 0) -> ("发送成功"=w4184:bool)  [unwired: 8 out]
                  }
                }
                n3111 = stacked-sequence {
                  tunnel: [w4169] -> w4160
                  frame #0 {
                    w4169 = TRUE ("控制1")
                    w4172 = FALSE ("写?")
                    n3112 = call <vilib>:"Set Busy.vi"("disable click? (T)"=FALSE) -> ()  [unwired: 3 in, 8 out]
                    n3113 = local write "写?"(w4172) -> ()
                    n3114 = global write "EV05全局变量1.vi" "写入超时"(w4172) -> ()
                    n3115 = local write "主从选择"(enum32{"主板", "从板"}."主板" ("主从选择")) -> ()
                    n3116 = local write "清BUFF"(FALSE ("清BUFF")) -> ()
                    n3117 = property on="保存版本信息" class="Bool (严格)"("Visible"=TRUE ("可见")) -> ()  [unwired: 2 in, 2 out]
                    n3118 = global write "EV05全局变量1.vi" "流控帧 2"(TRUE ("流控帧 2")) -> ()
                    n3119 = local write "控制1"(w4169) -> ()
                    n3120 = local write "消除"(TRUE ("消除")) -> ()
                    n3121 = global write "EV05全局变量1.vi" "流控帧"(FALSE ("流控帧")) -> ()
                  }
                }
                n3122 = case shown="真" w4162 {
                  tunnel: w4166 -> [w4186 w4191]
                  tunnel: w4165 -> [w4185 w4190]
                  tunnel: [w4186 w4188] -> w4164
                  tunnel: [w4185 w4187] -> w4163
                  tunnel: w4160 -> [_ _]
                  frame False {
                  }
                  frame True {
                    n3123 = Enqueue Element(queue=w4191, element="模块软件版本读取" ("元素"), error in (no error)=w4190) -> (queue out=w4188:refnum<queue>, error out=w4187:errorcluster)  [unwired: 2 out]
                  }
                }
              }
            }
          }
          event "保存版本信息": Value Change {
            n3124 = event-data() -> ("NewVal"=w4192:bool)  [unwired: 6 out]
            n3125 = case shown="真" w4192 {
              frame False {
              }
              frame True {
                n3126 = stacked-sequence {
                  seq-local: [w4196 _] -> [_ w4198]
                  seq-local: [w4195 _] -> [_ w4197]
                  frame #0 {
                    n3127 = call "请输入从板个数"() -> ("从板个数"=w4196:dbl, "确定"=w4195:bool)  [unwired: 17 in, 1 out]
                  }
                  frame #1 {
                    n3128 = case shown="真" w4197 {
                      tunnel: w4198 -> [_ w4201]
                      frame False {
                      }
                      frame True {
                        n3129 = call <vilib>:"Application Directory.vi"() -> ("Application Directory"=w4213:path)
                        n3130 = Build Path(base path=w4213, name or relative path="SaveData" ("名称或相对路径")) -> (appended path=w4211:path)
                        n3131 = local read "模块版本名称"() -> (w4206:string[][])
                        n3132 = local read "项目软件版本"() -> (w4203:string[])
                        n3133 = local read "模块版本值"() -> (w4205:string[][])
                        n3134 = local read "平台软件版本"() -> (w4202:string[])
                        n3135 = local read "模块个数"() -> (w4199:u8[])
                        n3136 = local read "硬件版本"() -> (w4204:string[])
                        n3137 = call "文件对话框3"("start path"=w4211, "prompt"="选择要保存数据的位置", "default name"="BMS版本信息.txt") -> ("selected path"=w4207:path, "cancelled"=w4208:bool)  [unwired: 9 in, 2 out]
                        n3138 = Increment(x=w4201) -> (x+1=w4200:dbl)
                        n3139 = for {
                          N: w4200 -> [_]
                          tunnel: w4208 -> [w4229]
                          tunnel: w4207 -> [w4228]
                          tunnel: w4206 -> [w4218] mode=indexing
                          tunnel: w4205 -> [w4216] mode=indexing
                          tunnel: w4204 -> [w4223] mode=indexing
                          tunnel: w4203 -> [w4222] mode=indexing
                          tunnel: w4202 -> [w4221] mode=indexing
                          tunnel: w4199 -> [w4214] mode=indexing
                          i -> [w4220]
                          w4226 = ""
                          w4233 = 0 ("索引")
                          n3140 = case shown="0, 默认" w4220 {
                            selector: w4220 -> [_ w4247]
                            tunnel: ["主板版本信息" w4248] -> w4238
                            tunnel: [FALSE TRUE] -> w4224
                            frame 0, Default {
                            }
                            frame 1.. {
                              n3141 = Number To Decimal String(number=w4247) -> (decimal integer string=w4246:string)  [unwired: 1 in]
                              n3142 = Concatenate Strings("从板", w4246, "版本信息") -> (w4248:string)
                            }
                          }
                          n3143 = Increment(x=w4214) -> (x+1=w4215:u8)
                          n3144 = Array Subset(array=w4218, length=w4215) -> (w4219:string[])  [unwired: 1 in]
                          n3145 = Array Subset(array=w4216, length=w4215) -> (w4217:string[])  [unwired: 1 in]
                          n3146 = Build Array(w4226, w4221, w4222, w4223, w4226) -> (w4232:string[])
                          n3147 = Build Array(w4238, "平台软件版本号", "项目软件版本号", "硬件版本号", "模块版本号") -> (w4234:string[])
                          n3148 = Insert Into Array(array=w4219, index=w4233, new element=w4234) -> (w4231:string[])
                          n3149 = Insert Into Array(array=w4217, index=w4233, new element=w4232) -> (w4230:string[])
                          n3150 = Build Array(w4231, w4230) -> (w4227:string[][])
                          n3151 = case shown="假" w4229 {
                            tunnel: w4228 -> [w4242 _]
                            tunnel: w4227 -> [w4241 _]
                            tunnel: w4224 -> [w4239 _]
                            frame False {
                              n3152 = call-poly <vilib>:"Write To Spreadsheet File.vi"("transpose? (no:F)"=TRUE, "append to file? (new file:F)"=w4239, "2D data"=w4241, "file path (dialog if empty)"=w4242) -> ()  [unwired: 4 in, 1 out]
                            }
                            frame True {
                            }
                          }
                        }
                      }
                    }
                  }
                }
              }
            }
          }
          event "单个写入": Value Change {
            n3153 = event-data() -> ("NewVal"=w4255:bool)  [unwired: 5 out]
            n3154 = case shown="真" w4255 {
              tunnel: w4254 -> [w4257 w4264]
              tunnel: w4253 -> [w4256 w4263]
              tunnel: [w4257 w4262] -> w4252
              tunnel: [w4256 w4261] -> w4251
              frame False {
              }
              frame True {
                w4259 = FALSE ("流控帧")
                w4258 = TRUE ("流控帧 2")
                n3155 = disable-structure shown="启用" {
                  disable-tunnel: [w4273 TRUE ("发送成功")] -> w4260
                  frame Disabled {
                    n3156 = local read "主从选择"() -> (w4265:enum32{"主板", "从板"})
                    n3157 = case shown="\"主板\", 默认" w4265 {
                      tunnel: [0.0 ("FUNC") w4275] -> w4270
                      frame "主板", Default {
                      }
                      frame "从板" {
                        n3158 = local read "从板号"() -> (w4275:u8)
                      }
                    }
                    n3159 = local read "设备索引号"() -> (w4267:u16)
                    n3160 = local read "CAN卡类型"() -> (w4268:u32)
                    n3161 = local read "CAN端口"() -> (w4266:u16)
                    n3162 = call "标定授权发送.vi"("CAN卡类型"=w4268, "解锁类型"=enum16{"读取", "写", "下载"}."写", "设备索引号"=w4267, "CAN端口"=w4266, "是否连接"=TRUE, "板选择"=0, "FUNC"=w4270) -> ("发送成功"=w4273:bool)  [unwired: 8 out]
                  }
                  frame Enabled {
                  }
                }
                n3163 = case shown="真" w4260 {
                  tunnel: w4264 -> [w4278 w4282]
                  tunnel: w4263 -> [w4277 w4281]
                  tunnel: [w4278 w4284] -> w4262
                  tunnel: [w4277 w4283] -> w4261
                  frame False {
                  }
                  frame True {
                    n3164 = Flush Queue(queue=w4282, error in (no error)=w4281) -> (queue out=w4280:refnum<queue>, error out=w4279:errorcluster)  [unwired: 1 out]
                    n3165 = Enqueue Element(queue=w4280, element="单个写入" ("元素"), error in (no error)=w4279) -> (queue out=w4284:refnum<queue>, error out=w4283:errorcluster)  [unwired: 2 out]
                  }
                }
                n3166 = global write "EV05全局变量1.vi" "读取超时"(w4259) -> ()
                n3167 = global write "EV05全局变量1.vi" "流控帧"(w4259) -> ()
                n3168 = local write "消除"(w4258) -> ()
                n3169 = local write "控制1"(w4258) -> ()
                n3170 = global write "EV05全局变量1.vi" "流控帧 2"(w4258) -> ()
                n3171 = local write "写?"(w4258) -> ()
              }
            }
          }
          event "全部写入": Value Change {
            n3172 = event-data() -> ("NewVal"=w4290:bool)  [unwired: 5 out]
            n3173 = case shown="真" w4290 {
              tunnel: w4289 -> [w4292 w4300]
              tunnel: w4288 -> [w4291 w4299]
              tunnel: [w4292 w4298] -> w4287
              tunnel: [w4291 w4297] -> w4286
              frame False {
              }
              frame True {
                w4294 = FALSE ("流控帧")
                w4293 = TRUE ("流控帧 2")
                n3174 = global read "EV05全局变量1.vi" "授权功能"() -> (w4295:bool)
                n3175 = case shown="真" w4295 {
                  tunnel: [TRUE ("发送成功") w4310] -> w4296
                  frame False {
                  }
                  frame True {
                    n3176 = local read "主从选择"() -> (w4302:enum32{"主板", "从板"})
